vi "Test ESP8266 UPD Server Write to Clients.vi"() -> ()   [LabVIEW 2014]
uses:
  <vilib>/LabVIEW Universal Transcriptor/LabVIEW to Arduino Transcriptor/Transcriptors/System API/Serial println string.vi
  <vilib>/LabVIEW Universal Transcriptor/ESP8266 WiFi Wrapper/ESP8266 WiFi Wrapper.lvlib
panel:
  out "Error Out":errorcluster
  in  "DNS address":u8[](array[numeric])=[0, 0, 0, 0]
  in  "IP address":u8[](array[numeric])=[192, 168, 0, 47]
  in  "Gateway":u8[](array[numeric])=[192, 168, 0, 1]
  in  "Subnet mask":u8[](array[numeric])=[255, 255, 255, 0]
  in  "Password":string="12345678"
  in  "SSID":string="ESP8266 Wifi UDP"
  in  "Listen Port":i16=8080
  in  "error in (no error)":errorcluster
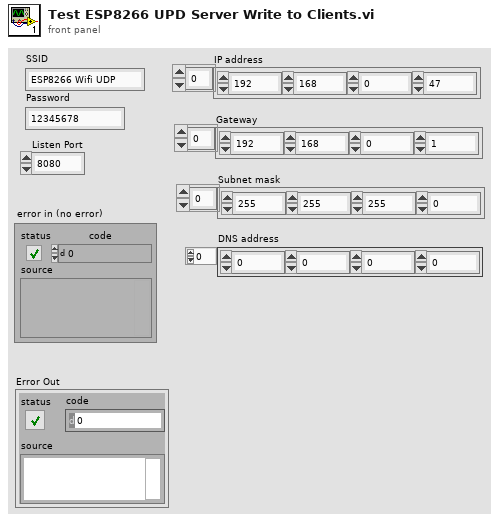
[diagram p1: front panel]
types:
  T1 = enum16{"WIFI_OFF", "WIFI_STA", "WIFI_AP", "WIFI_AP_STA"}
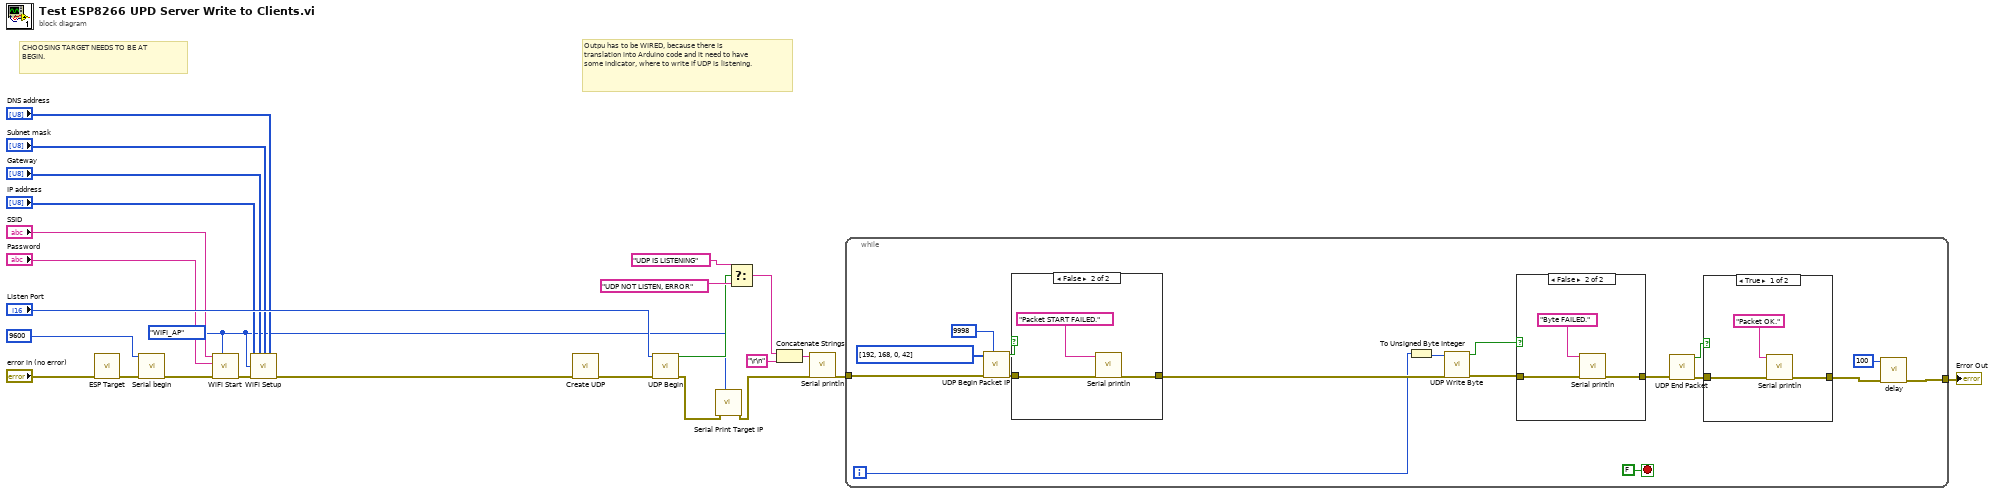
[diagram p0: block diagram]
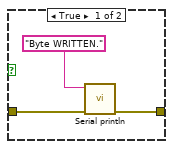
[diagram p2: hidden frame]
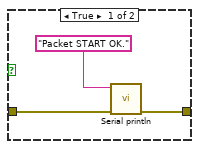
[diagram p3: hidden frame]
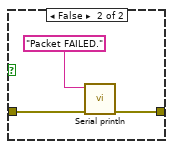
[diagram p4: hidden frame]
diagram:
  w2 = T1."WIFI_AP" ("WiFi Mode")
  # "Outpu has to be WIRED, because there is translation into Arduino code and it need to have some indicator, where to write if UDP is listening."
  # "CHOOSING TARGET NEEDS TO BE AT BEGIN."
  n1 = call <vilib>:"ESP Target.vi"("Error In"="error in (no error)") -> ("Error Out"=w24:errorcluster)  [unwired: 10 in]
  n2 = call <vilib>:"Serial begin.vi"("Error In"=w24, "speed (Bd)"=u32 9600 ("Speed")) -> ("Error Out"=w15:errorcluster)  [unwired: 9 in]
  n3 = call <vilib>:"WiFi Start.vi"("WiFi Mode"=w2, "Error In"=w15, "Password"="Password", "SSID"="SSID") -> ("Error Out"=w14:errorcluster)  [unwired: 7 in]
  n4 = call <vilib>:"WiFi Setup.vi"("IP address"="IP address", "Gateway address"="Gateway", "Subnet mask"="Subnet mask", "DNS address"="DNS address", "WiFi Mode"=w2, "Error In"=w14) -> ("Error Out"=w1:errorcluster)  [unwired: 9 in]
  n5 = call <vilib>:"Create UDP.vi"("Error In"=w1) -> ("Error Out"=w13:errorcluster)  [unwired: 10 in]
  n6 = call <vilib>:"UDP Begin.vi"("Error In"=w13, "Port"="Listen Port") -> ("Error Out"=w4:errorcluster, "Is listening?"=w9:bool)  [unwired: 8 in]
  n7 = call <vilib>:"Serial Print Target IP.vi"("WiFi Mode"=w2, "Error In"=w4) -> ("Error Out"=w3:errorcluster)  [unwired: 9 in]
  n8 = Select(t="UDP IS LISTENING", s=w9, f="UDP NOT LISTEN, ERROR") -> (s? t:f=w6:string)
  n9 = Concatenate Strings(w6, "\r\n") -> (w8:string)
  n10 = call-poly <vilib>:"Serial println.vi"("Error In"=w3, "string in"=w8) -> ("Error Out"=w12:errorcluster)  [unwired: 9 in]
  n11 = while {
    tunnel: w12 -> [w39]
    tunnel: [w40] -> w5
    i -> [w26]
    stop <- FALSE stop-if-true
    n12 = call <vilib>:"UDP Begin Packet IP.vi"("Port"=i16 9998, "Error In"=w39, "IP Address"=u8[] [192, 168, 0, 42]) -> ("Error Out"=w33:errorcluster, "Successful?"=w32:bool)  [unwired: 7 in]
    n13 = case shown="False" w32 {
      tunnel: w33 -> [w51 w54]
      tunnel: [w50 w53] -> w29
      frame True {
        n14 = call-poly <vilib>:"Serial println.vi"("Error In"=w51, "string in"="Packet START OK.") -> ("Error Out"=w50:errorcluster)  [unwired: 9 in]
      }
      frame False {
        n15 = call-poly <vilib>:"Serial println.vi"("Error In"=w54, "string in"="Packet START FAILED.") -> ("Error Out"=w53:errorcluster)  [unwired: 9 in]
      }
    }
    n16 = To Unsigned Byte Integer(number=w26) -> (unsigned 8bit integer=w27:u8)
    n17 = call <vilib>:"UDP Write Byte.vi"("Error In"=w29, "Byte to write"=w27) -> ("Error Out"=w30:errorcluster, "Byte written?"=w28:bool)  [unwired: 8 in]
    n18 = case shown="False" w28 {
      tunnel: w30 -> [w45 w48]
      tunnel: [w44 w47] -> w31
      frame True {
        n19 = call-poly <vilib>:"Serial println.vi"("Error In"=w45, "string in"="Byte WRITTEN.") -> ("Error Out"=w44:errorcluster)  [unwired: 9 in]
      }
      frame False {
        n20 = call-poly <vilib>:"Serial println.vi"("Error In"=w48, "string in"="Byte FAILED.") -> ("Error Out"=w47:errorcluster)  [unwired: 9 in]
      }
    }
    n21 = call <vilib>:"UDP End Packet.vi"("Error In"=w31) -> ("Error Out"=w37:errorcluster, "Successful?"=w35:bool)  [unwired: 9 in]
    n22 = case shown="True" w35 {
      tunnel: w37 -> [w57 w60]
      tunnel: [w56 w59] -> w36
      frame True {
        n23 = call-poly <vilib>:"Serial println.vi"("Error In"=w57, "string in"="Packet OK.") -> ("Error Out"=w56:errorcluster)  [unwired: 9 in]
      }
      frame False {
        n24 = call-poly <vilib>:"Serial println.vi"("Error In"=w60, "string in"="Packet FAILED.") -> ("Error Out"=w59:errorcluster)  [unwired: 9 in]
      }
    }
    n25 = call <vilib>:"delay.vi"("Error In"=w36, "time (ms)"=100) -> ("Error Out"=w40:errorcluster)  [unwired: 9 in]
  }
  "Error Out" <- w5
